vi "ITC Reply to PGSQL.vi"(8 "error in (no error)":errorcluster, 10 "Response":T1, 11 "Instrument.1820 in":refnum<class "Instrument.Oxford1820.lvclass">) -> (0 "error out":errorcluster, 3 "Instrument.1820 out":refnum<class "Instrument.Oxford1820.lvclass">)   [LabVIEW 2019, in "Instrument.Oxford1820.lvclass"]
uses:
  Instrument.Oxford1820.lvclass
  <instrlib>/Mercury iXX/Public/Controls/Response String.ctl
  C:/Program Files (x86)/National Instruments/LabVIEW 2019/user.lib/LevyLab/Instrument Framework/Instrument/Instrument.lvclass
  <userlib>/LevyLab/Instrument Framework/Instrument/Instrument.lvclass
  <instrlib>/Mercury iXX/Mercury iXX.lvlib
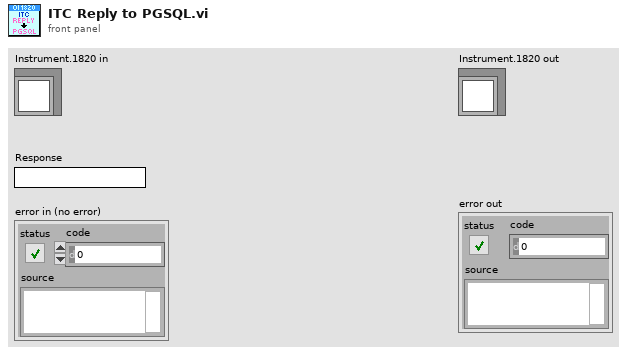
[diagram p1: front panel]
types:
  T1 = typedef "Mercury iXX.lvlib/Response String.ctl" = string
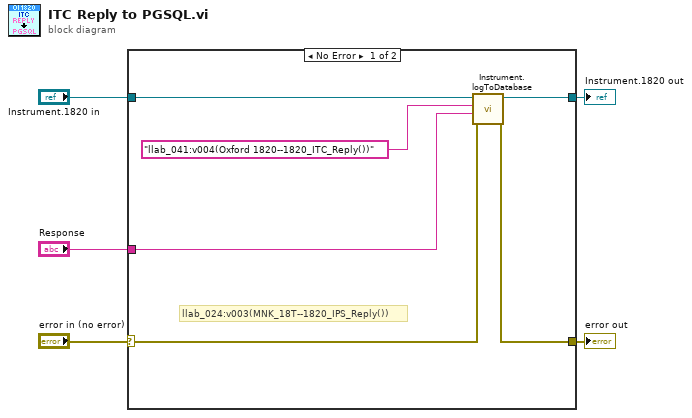
[diagram p0: block diagram]
diagram:
  n1 = case shown="No Error" "error in (no error)" {
    selector: "error in (no error)" -> [w10 w12]
    tunnel: "Response" -> [w11 _]
    tunnel: [w9 w12] -> w4
    tunnel: "Instrument.1820 in" -> [w8 w13]
    tunnel: [w7 w13] -> w1
    frame No Error {
      # "llab_024:v003(MNK_18T--1820_IPS_Reply())"
      n2 = call <userlib>:"Instrument.logToDatabase.vi"("error in (no error)"=w10, "Data"=w11, "Paths"="llab_041:v004(Oxford 1820--1820_ITC_Reply())" ("variable"), "Instrument"=w8) -> ("error out"=w9:errorcluster, "Instrument out"=w7:refnum<class "Instrument.Oxford1820.lvclass">)  [unwired: 6 in]
    }
    frame Error {
    }
  }
  "error out" <- w4
  "Instrument.1820 out" <- w1
